vi "dfd_WordLen to SHFT.vi"(1 "wl":i16) -> (0 "SHFT":i16)   [LabVIEW 2017, in "NI_DigFilter_FXP.lvlib"]
uses:
  <vilib>/addons/Digital Filter Design/NI_DigFilter_FXP.lvlib
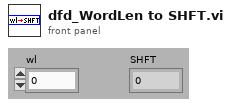
[diagram p1: front panel]
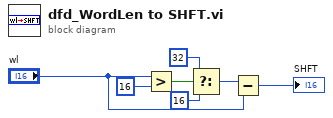
[diagram p0: block diagram]
diagram:
  n1 = Greater?(x="wl", y=i16 16) -> (0:w2:bool)
  n2 = Select(t=i16 32 ("y"), s=w2, f=i16 16) -> (s? t:f=w5:i16)
  n3 = Subtract(x=w5, y="wl") -> (x-y=→"SHFT":i16)
